vi "Control_Pump_Valves.vi"(3 "Set state:":bool, 5 "Device":T1=enum."V7") -> (0 "Good Reply":bool, 2 "Comment":string)   [LabVIEW 2010]
uses:
  Valve_Pump.ctl
  ADAM Client/Sub VIs/ADAM Controls/Address.ctl
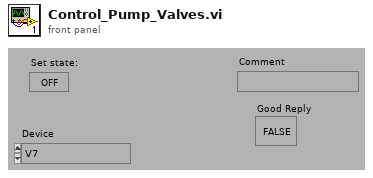
[diagram p1: front panel]
types:
  T1 = typedef "Valve_Pump.ctl" = enum16{"Main Rack Power", "Pump Power", "Valve Power", "V4", "V5", "V6", "V7", "V8", "V9", "V10", "V11", "V12", "V13", "V14", "V15", "V18", "V19", "V20", "V21", "V22", "V23", "V24", "V25", "V26", "V27", "V28", "V29", "V30", "V31", "V32", "V33", "V34", "Spare", "V42", "V37", "Pump A", "Pump B", "Pump C", "Pump D"}
  T2 = typedef "Address.ctl" = cluster{"Main":i32, "Ch.":i32, "Sub":i32, "Port Name":string}
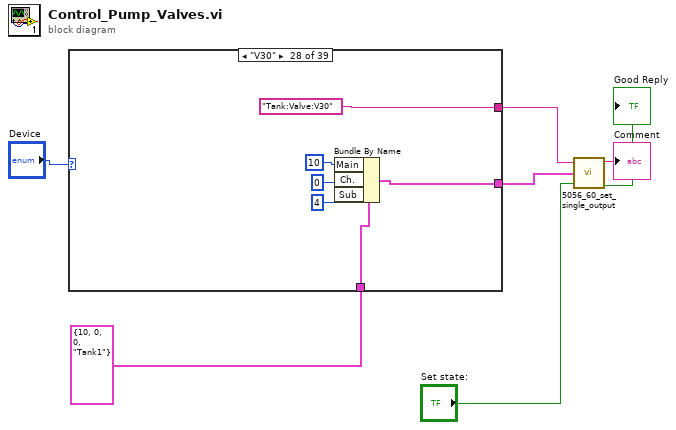
[diagram p0: block diagram]
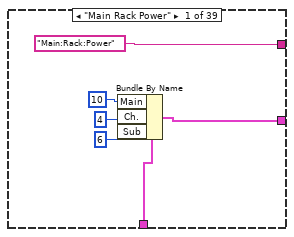
[diagram p2: hidden frame]
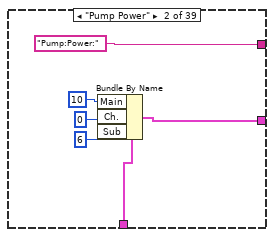
[diagram p3: hidden frame]
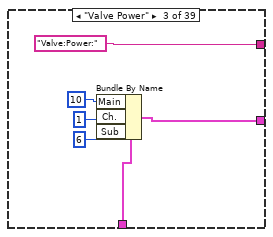
[diagram p4: hidden frame]
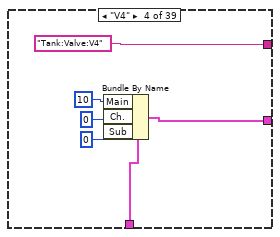
[diagram p5: hidden frame]
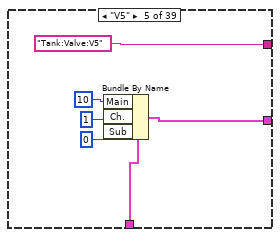
[diagram p6: hidden frame]
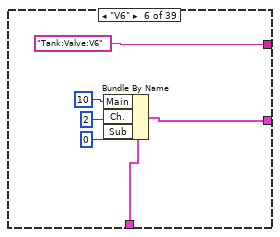
[diagram p7: hidden frame]
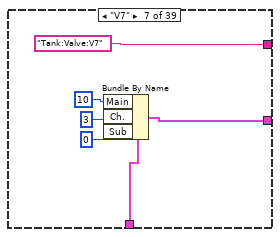
[diagram p8: hidden frame]
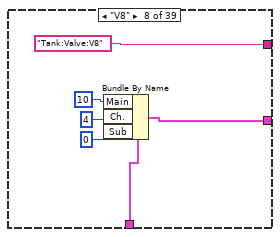
[diagram p9: hidden frame]
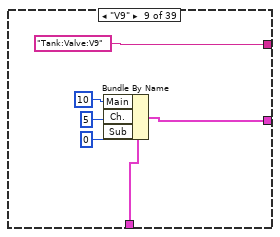
[diagram p10: hidden frame]
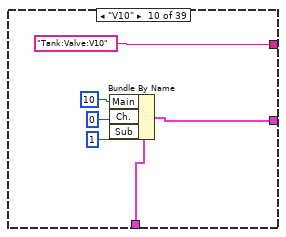
[diagram p11: hidden frame]
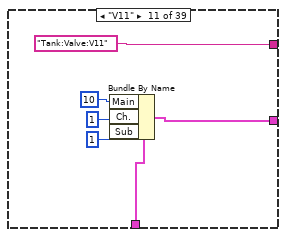
[diagram p12: hidden frame]
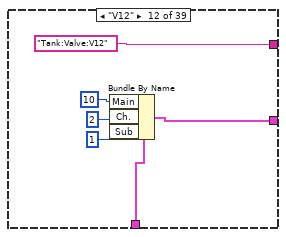
[diagram p13: hidden frame]
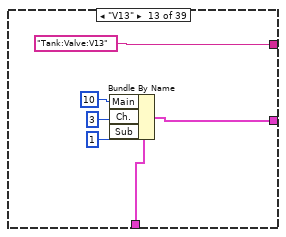
[diagram p14: hidden frame]
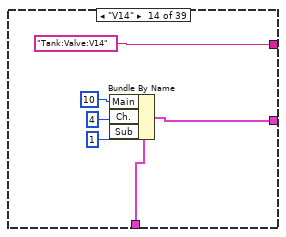
[diagram p15: hidden frame]
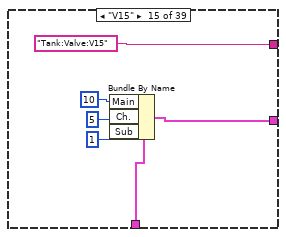
[diagram p16: hidden frame]
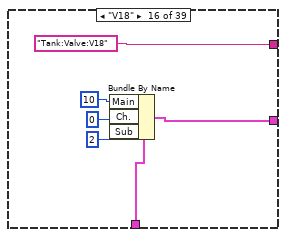
[diagram p17: hidden frame]
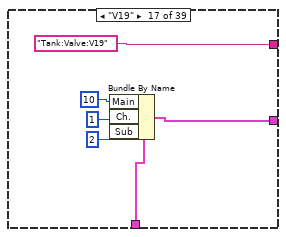
[diagram p18: hidden frame]
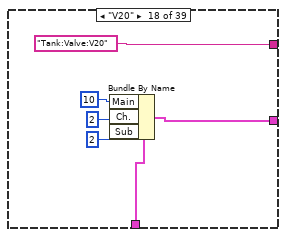
[diagram p19: hidden frame]
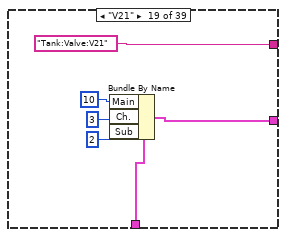
[diagram p20: hidden frame]
diagram:
  n1 = case shown="\"V30\"" "Device" {
    tunnel: T2 {"Main"=10, "Ch."=0, "Sub"=0, "Port Name"="Tank1"} ("Address (all reqd.)") -> [w13 w19 w25 w31 w37 w43 w49 w55 w61 w67 w73 w79 w85 w91 w97 w103 w109 w115 w121 w127 w133 w139 w145 w151 w157 w163 w169 w175 w181 w187 w193 w199 w205 w211 w217 w223 w229 w235 w241]
    tunnel: [w9 w15 w21 w27 w33 w39 w45 w51 w57 w63 w69 w75 w81 w87 w93 w99 w105 w111 w117 w123 w129 w135 w141 w147 w153 w159 w165 w171 w177 w183 w189 w195 w201 w207 w213 w219 w225 w231 w237] -> w5
    tunnel: ["Main:Rack:Power" ("Channel Name") "Pump:Power:" ("Channel Name") "Valve:Power:" ("Channel Name") "Tank:Valve:V4" ("Channel Name") "Tank:Valve:V5" ("Channel Name") "Tank:Valve:V6" ("Channel Name") "Tank:Valve:V7" ("Channel Name") "Tank:Valve:V8" ("Channel Name") "Tank:Valve:V9" ("Channel Name") "Tank:Valve:V10" ("Channel Name") "Tank:Valve:V11" ("Channel Name") "Tank:Valve:V12" ("Channel Name") "Tank:Valve:V13" ("Channel Name") "Tank:Valve:V14" ("Channel Name") "Tank:Valve:V15" ("Channel Name") "Tank:Valve:V18" ("Channel Name") "Tank:Valve:V19" ("Channel Name") "Tank:Valve:V20" ("Channel Name") "Tank:Valve:V21" ("Channel Name") "Tank:Valve:V22" ("Channel Name") "Tank:Valve:V23" ("Channel Name") "Tank:Valve:V24" ("Channel Name") "Tank:Valve:V25" ("Channel Name") "Tank:Valve:V26" ("Channel Name") "Tank:Valve:V27" ("Channel Name") "Tank:Valve:V28" ("Channel Name") "Tank:Valve:V29" ("Channel Name") "Tank:Valve:V30" ("Channel Name") "Tank:Valve:V31" ("Channel Name") "Tank:Valve:V32" ("Channel Name") "Tank:Valve:V33" ("Channel Name") "Tank:Valve:V34" ("Channel Name") "Tank:Valve:V35" ("Channel Name") "Tank:Valve:V42" ("Channel Name") "Tank:Valve:V37" ("Channel Name") "Tank:Valve:Pump A" ("Channel Name") "Tank:Valve:Pump B" ("Channel Name") "Tank:Valve:Pump C" ("Channel Name") "Tank:Valve:Pump D" ("Channel Name")] -> w4
    frame "Main Rack Power" {
      n2 = Bundle By Name(cluster=w13, "Main"=10, "Ch."=4, "Sub"=6) -> (w9:T2)
    }
    frame "Pump Power" {
      n3 = Bundle By Name(cluster=w19, "Main"=10, "Ch."=0, "Sub"=6) -> (w15:T2)
    }
    frame "Valve Power" {
      n4 = Bundle By Name(cluster=w25, "Main"=10, "Ch."=1, "Sub"=6) -> (w21:T2)
    }
    frame "V4" {
      n5 = Bundle By Name(cluster=w31, "Main"=10, "Ch."=0, "Sub"=0) -> (w27:T2)
    }
    frame "V5" {
      n6 = Bundle By Name(cluster=w37, "Main"=10, "Ch."=1, "Sub"=0) -> (w33:T2)
    }
    frame "V6" {
      n7 = Bundle By Name(cluster=w43, "Main"=10, "Ch."=2, "Sub"=0) -> (w39:T2)
    }
    frame "V7" {
      n8 = Bundle By Name(cluster=w49, "Main"=10, "Ch."=3, "Sub"=0) -> (w45:T2)
    }
    frame "V8" {
      n9 = Bundle By Name(cluster=w55, "Main"=10, "Ch."=4, "Sub"=0) -> (w51:T2)
    }
    frame "V9" {
      n10 = Bundle By Name(cluster=w61, "Main"=10, "Ch."=5, "Sub"=0) -> (w57:T2)
    }
    frame "V10" {
      n11 = Bundle By Name(cluster=w67, "Main"=10, "Ch."=0, "Sub"=1) -> (w63:T2)
    }
    frame "V11" {
      n12 = Bundle By Name(cluster=w73, "Main"=10, "Ch."=1, "Sub"=1) -> (w69:T2)
    }
    frame "V12" {
      n13 = Bundle By Name(cluster=w79, "Main"=10, "Ch."=2, "Sub"=1) -> (w75:T2)
    }
    frame "V13" {
      n14 = Bundle By Name(cluster=w85, "Main"=10, "Ch."=3, "Sub"=1) -> (w81:T2)
    }
    frame "V14" {
      n15 = Bundle By Name(cluster=w91, "Main"=10, "Ch."=4, "Sub"=1) -> (w87:T2)
    }
    frame "V15" {
      n16 = Bundle By Name(cluster=w97, "Main"=10, "Ch."=5, "Sub"=1) -> (w93:T2)
    }
    frame "V18" {
      n17 = Bundle By Name(cluster=w103, "Main"=10, "Ch."=0, "Sub"=2) -> (w99:T2)
    }
    frame "V19" {
      n18 = Bundle By Name(cluster=w109, "Main"=10, "Ch."=1, "Sub"=2) -> (w105:T2)
    }
    frame "V20" {
      n19 = Bundle By Name(cluster=w115, "Main"=10, "Ch."=2, "Sub"=2) -> (w111:T2)
    }
    frame "V21" {
      n20 = Bundle By Name(cluster=w121, "Main"=10, "Ch."=3, "Sub"=2) -> (w117:T2)
    }
    frame "V22" {
      n21 = Bundle By Name(cluster=w127, "Main"=10, "Ch."=4, "Sub"=2) -> (w123:T2)
    }
    frame "V23" {
      n22 = Bundle By Name(cluster=w133, "Main"=10, "Ch."=5, "Sub"=2) -> (w129:T2)
    }
    frame "V24" {
      n23 = Bundle By Name(cluster=w139, "Main"=10, "Ch."=0, "Sub"=3) -> (w135:T2)
    }
    frame "V25" {
      n24 = Bundle By Name(cluster=w145, "Main"=10, "Ch."=1, "Sub"=3) -> (w141:T2)
    }
    frame "V26" {
      n25 = Bundle By Name(cluster=w151, "Main"=10, "Ch."=2, "Sub"=3) -> (w147:T2)
    }
    frame "V27" {
      n26 = Bundle By Name(cluster=w157, "Main"=10, "Ch."=3, "Sub"=3) -> (w153:T2)
    }
    frame "V28" {
      n27 = Bundle By Name(cluster=w163, "Main"=10, "Ch."=4, "Sub"=3) -> (w159:T2)
    }
    frame "V29" {
      n28 = Bundle By Name(cluster=w169, "Main"=10, "Ch."=5, "Sub"=3) -> (w165:T2)
    }
    frame "V30" {
      n29 = Bundle By Name(cluster=w175, "Main"=10, "Ch."=0, "Sub"=4) -> (w171:T2)
    }
    frame "V31" {
      n30 = Bundle By Name(cluster=w181, "Main"=10, "Ch."=1, "Sub"=4) -> (w177:T2)
    }
    frame "V32" {
      n31 = Bundle By Name(cluster=w187, "Main"=10, "Ch."=2, "Sub"=4) -> (w183:T2)
    }
    frame "V33" {
      n32 = Bundle By Name(cluster=w193, "Main"=10, "Ch."=3, "Sub"=4) -> (w189:T2)
    }
    frame "V34" {
      n33 = Bundle By Name(cluster=w199, "Main"=10, "Ch."=4, "Sub"=4) -> (w195:T2)
    }
    frame "Spare" {
      n34 = Bundle By Name(cluster=w205, "Main"=10, "Ch."=4, "Sub"=4) -> (w201:T2)
    }
    frame "V42" {
      n35 = Bundle By Name(cluster=w211, "Main"=10, "Ch."=5, "Sub"=4) -> (w207:T2)
    }
    frame "V37" {
      n36 = Bundle By Name(cluster=w217, "Main"=10, "Ch."=0, "Sub"=6) -> (w213:T2)
    }
    frame "Pump A" {
      n37 = Bundle By Name(cluster=w223, "Main"=10, "Ch."=0, "Sub"=5) -> (w219:T2)
    }
    frame "Pump B" {
      n38 = Bundle By Name(cluster=w229, "Main"=10, "Ch."=1, "Sub"=5) -> (w225:T2)
    }
    frame "Pump C" {
      n39 = Bundle By Name(cluster=w235, "Main"=10, "Ch."=2, "Sub"=5) -> (w231:T2)
    }
    frame "Pump D" {
      n40 = Bundle By Name(cluster=w241, "Main"=10, "Ch."=3, "Sub"=5) -> (w237:T2)
    }
  }
  n41 = call "5056_60_set_single_output.vi"("Channel Name"=w4, "Address (all reqd.)"=w5, "Set state:"="Set state:") -> ("Comment"=→"Comment":string, "Good Reply"=→"Good Reply":bool)  [unwired: 2 in]
